vi "Type.vi"(11 "Read Config File in":refnum<class "Read Config File.lvclass">) -> (2 "Name":string)   [LabVIEW 2025, in "Config Library.lvlib" / "Read Config File.lvclass"]
uses:
  Read Config File.lvclass
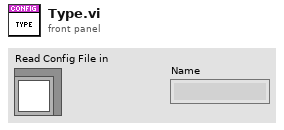
[diagram p1: front panel]
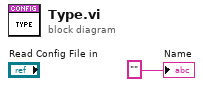
[diagram p0: block diagram]
diagram:
  "Name" <- ""
